vi "string_basics.vi"() -> ()   [LabVIEW 2020]
panel:
  out "number of replacements":i32
  out "replaced substring":string
  out "result string 2":string
  out "result string":string
  out "concatenated string":string
  in  "Lenght":dbl
  in  "Offset":dbl
  out "trimmed string":string
  out "all lower case string":string
  out "all upper case string":string
  out "length":i32
  in  "C":string
  in  "B":string
  in  "A":string
  # "INPUT DATA"
  # "STRING BASICS"
  # "REPLACE"
  # "SEARCH AND REPLACE"
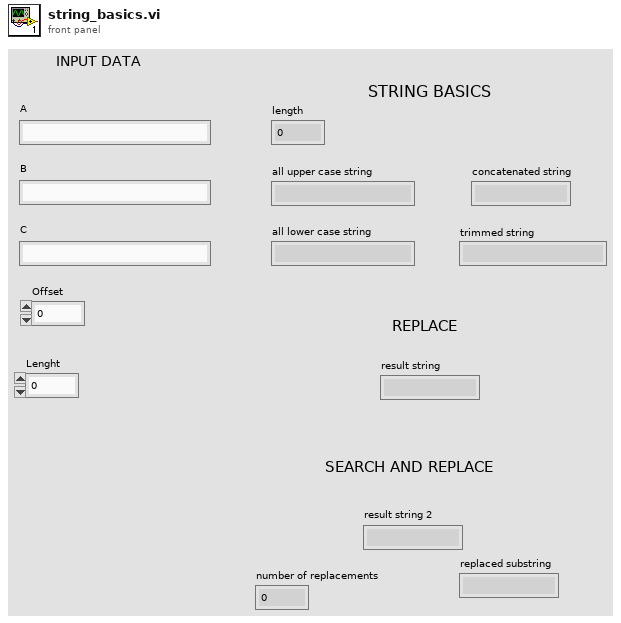
[diagram p1: front panel]
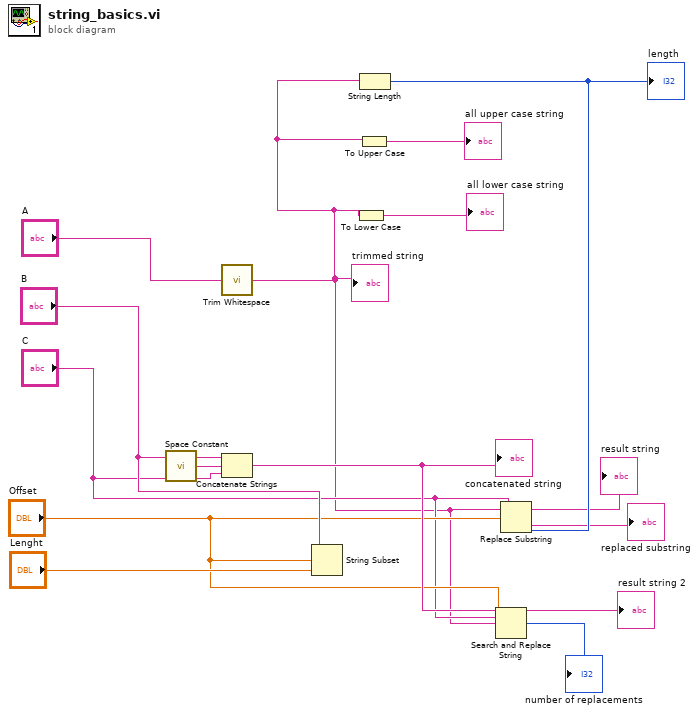
[diagram p0: block diagram]
diagram:
  n1 = call <vilib>:"Space Constant.vi"() -> ("String"=w3:string)
  n2 = call <vilib>:"Trim Whitespace.vi"("string"="A") -> ("trimmed string"=w1:string)  [unwired: 1 in]
  "trimmed string" <- w1
  n3 = Concatenate Strings "Concatenate Strings"("B", w3, "C") -> (w10:string)
  "concatenated string" <- w10
  n4 = String Subset(string="B", offset (0)="Offset", length (rest)="Lenght") -> ()  [unwired: 1 out]
  n5 = To Lower Case(string=w1) -> (all lower case string=→"all lower case string":string)
  n6 = To Upper Case(1:w1) -> (0:→"all upper case string":string)
  n7 = String Length(string=w1) -> (length=w11:i32)
  "length" <- w11
  n8 = Search and Replace String(input string=w10, search string="C", replace string=w1, offset="Offset") -> (result string=→"result string 2":string, number of replacements=→"number of replacements":i32)  [unwired: 4 in, 2 out]
  n9 = Replace Substring(2:w11, 3:"Offset", 4:w1, 5:"C") -> (0:→"replaced substring":string, 1:→"result string":string)
